vi "Vision Inspection Example.vi"(4 "Thread No.":u32, 5 "ProgramRef":refnum<vi>, 6 "Thread Mod Recive":refnum<queue>[](array[refnum]), 7 "ThreadsQueue":refnum<queue>[](array[refnum]), 8 "ThreadInfoIN":T1, 10 "StackIn":cluster{"Program":i32, "Prog Index":i32}[](array[cluster]), 11 "PrameterS":string) -> (0 "ThreadInfoOUT":T1, 2 "StackOut":cluster{"Program":i32, "Prog Index":i32}[](array[cluster]), 3 "ErrorCode":string)   [LabVIEW 2020]
uses:
  <vilib>/vision/Measure.llb/Edge Options.ctl
  <vilib>/vision/Measure.llb/Edge Polarity.ctl
  <vilib>/vision/Image Controls.llb/IMAQ Image.ctl
  <vilib>/vision/NI_Vision_Development_Module.lvlib
panel:
  in  "ResetPattern?":bool=TRUE
  out "DeltaAngle":sgl
  out "DeltaXY":cluster{"X":sgl, "Y":sgl}
  out "Angle":sgl=-46.475883
  out "CenterDL":cluster{"X":sgl, "Y":sgl}
  out "CenterUR":cluster{"X":sgl, "Y":sgl}
  in  "IMAQ?":bool=TRUE
  out "ROI Offset":cluster{"x":sgl, "y":sgl}
  out "FindCenter?":bool
  out "CenterPattern":T2(plugin-control)
  out "Pattern":T2(plugin-control)
  in  "SettingData":T5 {"FindCircleConfig"."Search  Direction" items=["Outside to Inside", "Inside to Outside"]; "FindCircleConfig"."Edge Options"."Edge Polarity" items=["All Edges", "Rising Edges", "Falling Edges"]; "FindCircleConfig"."Edge Options"."Minimum Edge Strength" format="%.2f"; "FindCircleConfig"."Edge Options"."Width" step=2; "FindCircleConfig"."Edge Options"."Kernel Size" step=2; "Range"."Maximum" format="%.2f"; "Range"."Minimum" format="%.2f"; "PatternCenter"."y" format="%.2f"; "PatternCenter"."x" format="%.2f"; "Algorithm" items=["All", "Low Discrepancy Sampling", "Grayscale Value Pyramid", "Gradients Pyramid"]}
  out "Test":T2(plugin-control)
  in  "Operation":enum16{"Setting", "Inspect"}(ring)=enum."Inspect"
  in  "ImagePath":path=path "D:/Project/V-KeyBoard Link Check/G3.png"
  # "ROI[0]: FindCenter"
  # "ROI[1]: Gap_up1"
  # "ROI[2]: Gap_up2"
  # "ROI[3]: Link_In1"
  # "ROI[4]: Link_In2"
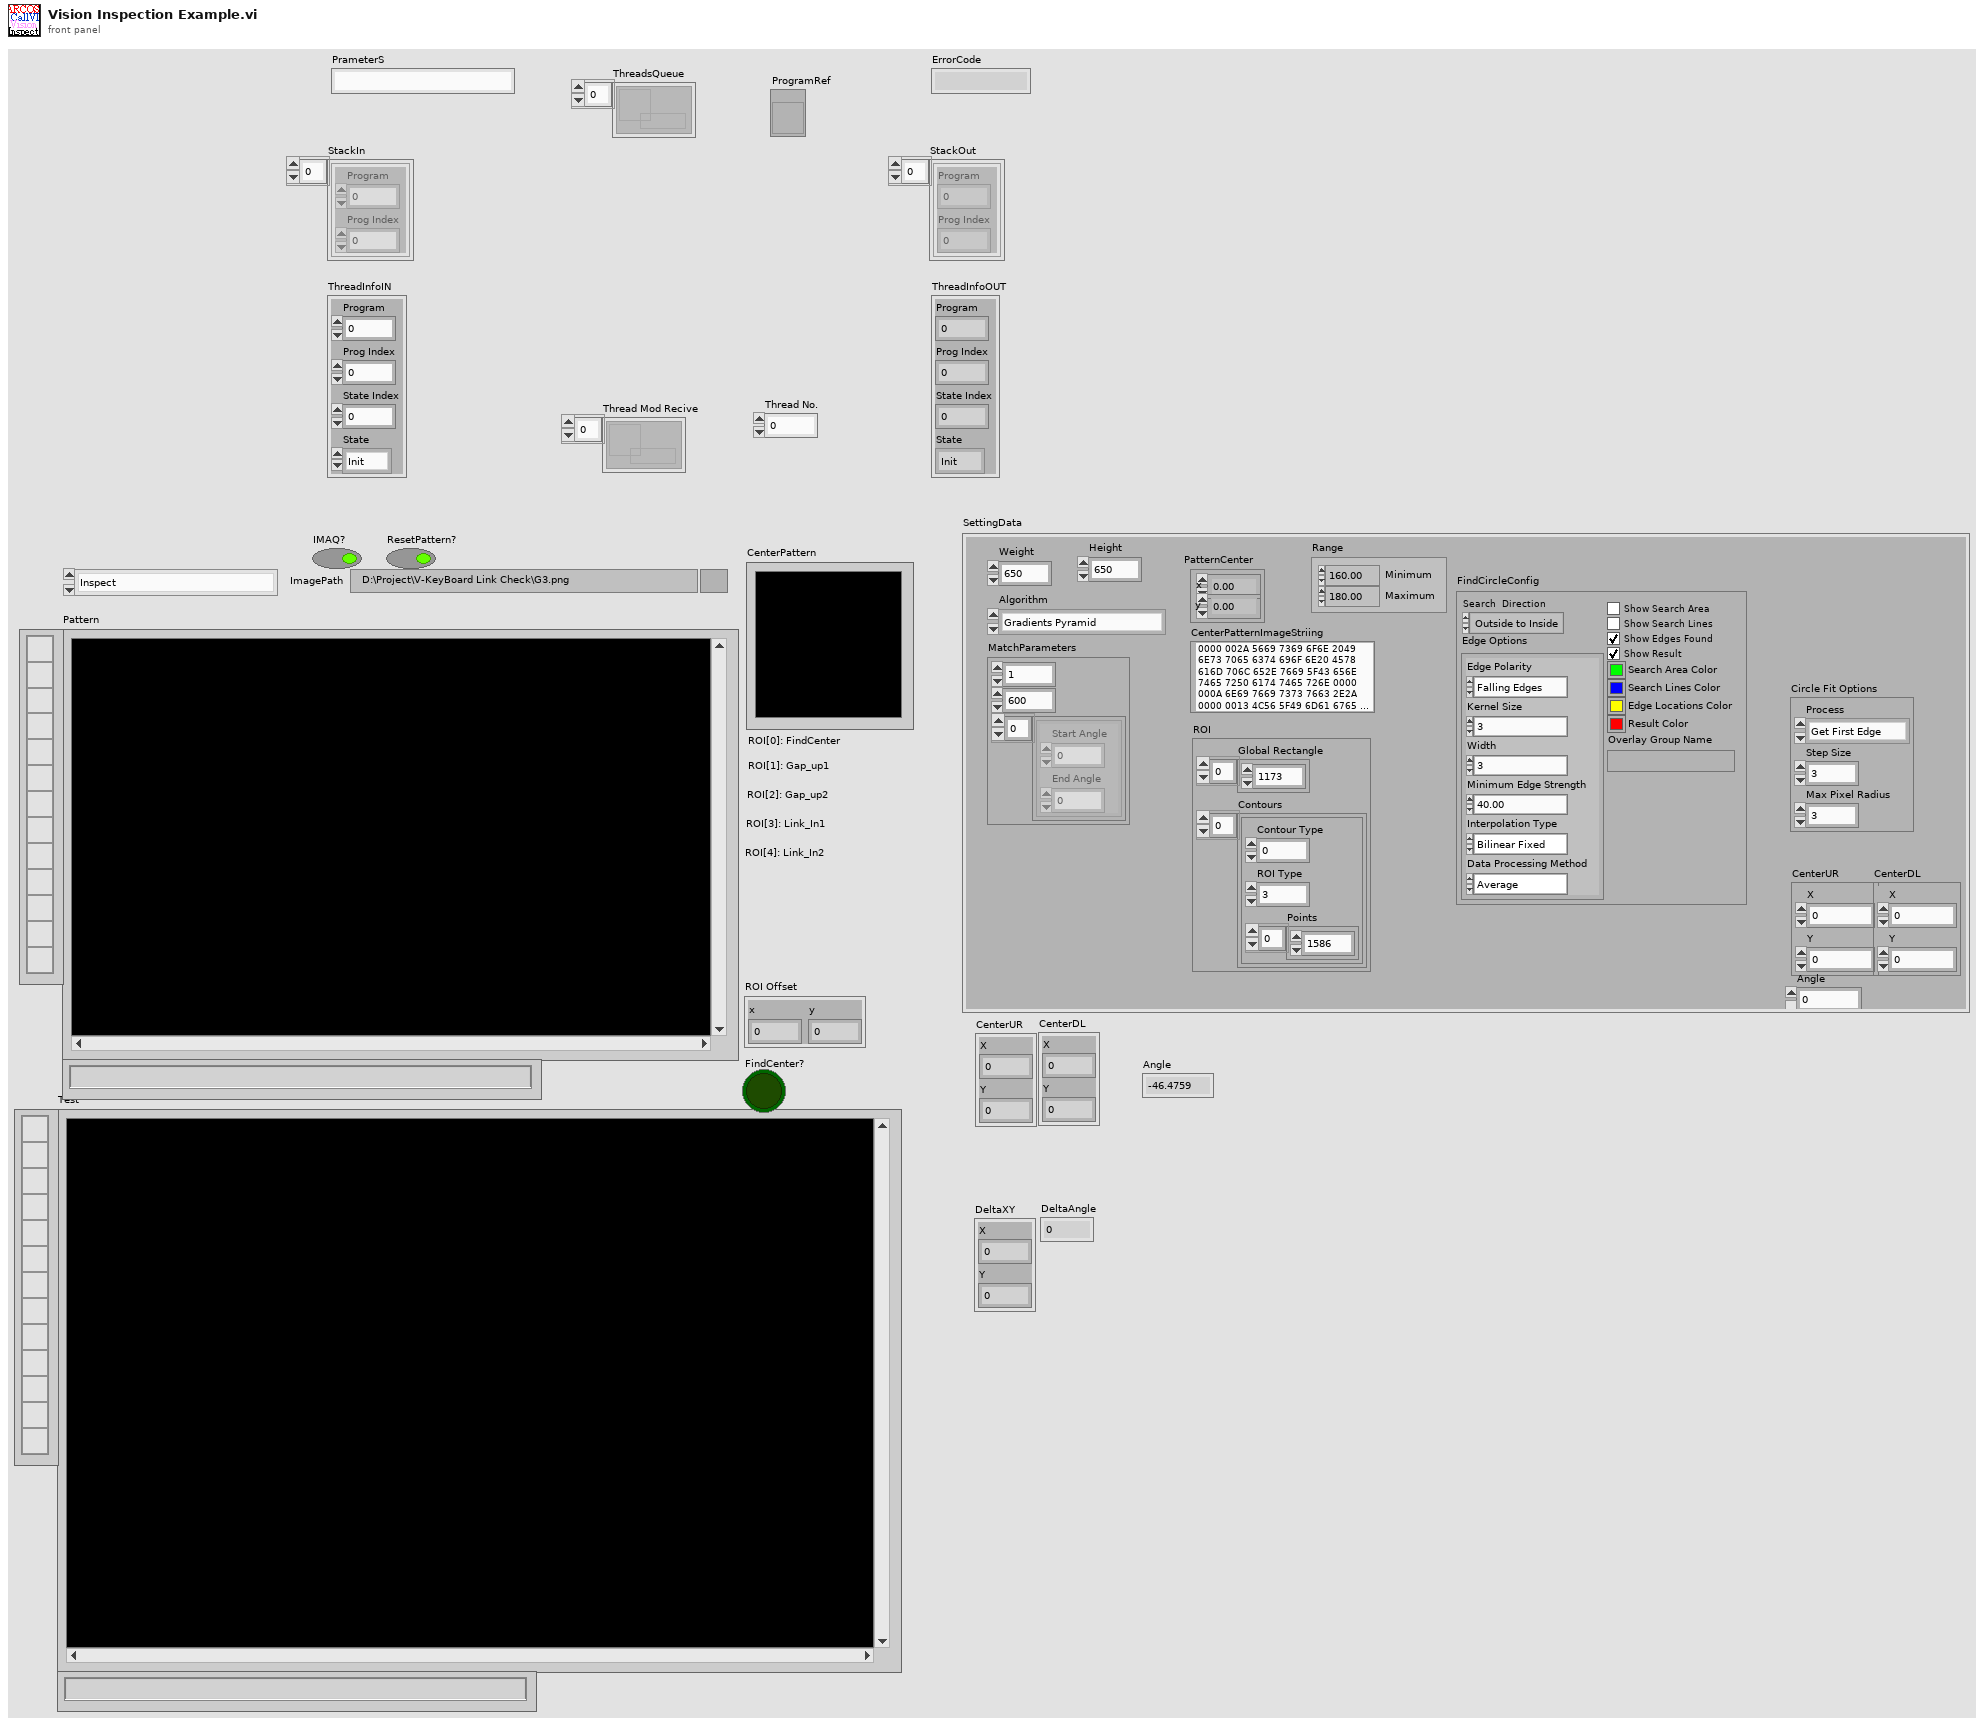
[diagram p1: front panel]
types:
  T1 = cluster{"Program":i32, "Prog Index":i32, "State Index":i32, "State":enum16{"Init", "Idle", "Auto Start", "Auto Running", "Step Start", "Step Running", "Suspend", "Restart", "Stop", "Reset"}}
  T2 = typedef "IMAQ Image.ctl" = refnum<image>
  T3 = typedef "Edge Options.ctl" = cluster{"Edge Polarity":T4, "Kernel Size":u32, "Width":u32, "Minimum Edge Strength":sgl, "Interpolation Type":enum32{"Zero Order", "Bilinear", "Quadratic", "Cubic", "Bilinear Fixed"}, "Data Processing Method":enum32{"Average", "Median"}}
  T4 = typedef "Edge Polarity.ctl" = u32
  T5 = cluster{"Weight":i32, "Height":i32, "MatchParameters":cluster{"Number of Matches Requested":i32, "Minimum Match Score":sgl, "Angle Ranges":cluster{"Start Angle":sgl, "End Angle":sgl}[]}, "Algorithm":i32, "CenterPatternImageStriing":string, "PatternCenter":cluster{"x":sgl, "y":sgl}, "ROI":cluster{"Global Rectangle":i32[], "Contours":cluster{"Contour Type":u32, "ROI Type":u32, "Points":i32[]}[]}, "Range":cluster{"Minimum":sgl, "Maximum":sgl}, "FindCircleConfig":cluster{"Search  Direction":u32, "Edge Options":T3, "Show Search Area":bool, "Show Search Lines":bool, "Show Edges Found":bool, "Show Result":bool, "Search Area Color":u32, "Search Lines Color":u32, "Edge Locations Color":u32, "Result Color":u32, "Overlay Group Name":string}, "Circle Fit Options":cluster{"Process":enum16{"Get First Edge", "Get First + Last Edge", "Get All Edges", "Get Best Edge"}, "Step Size":dbl, "Max Pixel Radius":i32}, "CenterUR":cluster{"X":sgl, "Y":sgl}, "CenterDL":cluster{"X":sgl, "Y":sgl}, "Angle":sgl}
  T6 = typedef "Image Type" = u32
  T7 = cluster{"Number of Matches Requested":i32, "Minimum Match Score":sgl, "Angle Ranges":cluster{"Start Angle":sgl, "End Angle":sgl}[]}
  T8 = cluster{"Search  Direction":u32, "Edge Options":T3, "Show Search Area":bool, "Show Search Lines":bool, "Show Edges Found":bool, "Show Result":bool, "Search Area Color":u32, "Search Lines Color":u32, "Edge Locations Color":u32, "Result Color":u32, "Overlay Group Name":string}
  T9 = cluster{"Process":enum16{"Get First Edge", "Get First + Last Edge", "Get All Edges", "Get Best Edge"}, "Step Size":dbl, "Max Pixel Radius":i32}
  T10 = cluster{"Global Rectangle":i32[], "Contours":cluster{"Contour Type":u32, "ROI Type":u32, "Points":i32[]}[]}
  T11 = cluster{"Contour Type":u32, "ROI Type":u32, "Points":i32[]}[]
  T12 = cluster{"Contour Type":u32, "ROI Type":u32, "Points":i32[]}
  T13 = cluster{"Position":cluster{"x":sgl, "y":sgl}, "Angle":sgl, "Scale":sgl, "Score":sgl, "Bounding Box":cluster{"x":sgl, "y":sgl}[]}[]
  T14 = cluster{"Position":cluster{"x":sgl, "y":sgl}, "Angle":sgl, "Scale":sgl, "Score":sgl, "Bounding Box":cluster{"x":sgl, "y":sgl}[]}
  T15 = cluster{"Center (Pixels)":cluster{"X":sgl, "Y":sgl}, "Radius (Pixels)":dbl, "Center (Real-World)":cluster{"X":sgl, "Y":sgl}, "Radius (Real-World)":dbl, "Roundness (Real-World)":dbl, "Average Strength":dbl, "Average SNR (dB)":dbl}
  T16 = cluster{"Origin":cluster{"X":sgl, "Y":sgl}, "Angle (deg)":sgl, "Axis Reference":u32}
  T17 = cluster{"ID":enum32{"External", "Internal"}, "Type":u32, "Coordinates":i32[]}[]
  T18 = cluster{"ID":enum32{"External", "Internal"}, "Type":u32, "Coordinates":i32[]}
  T19 = typedef "ROI Descriptor" = cluster{"Global Rectangle":i32[], "Contours":cluster{"ID":enum32{"External", "Internal"}, "Type":u32, "Coordinates":i32[]}[]}
  T20 = enum16{"Init", "Idle", "Auto Start", "Auto Running", "Step Start", "Step Running", "Suspend", "Restart", "Stop", "Reset"}
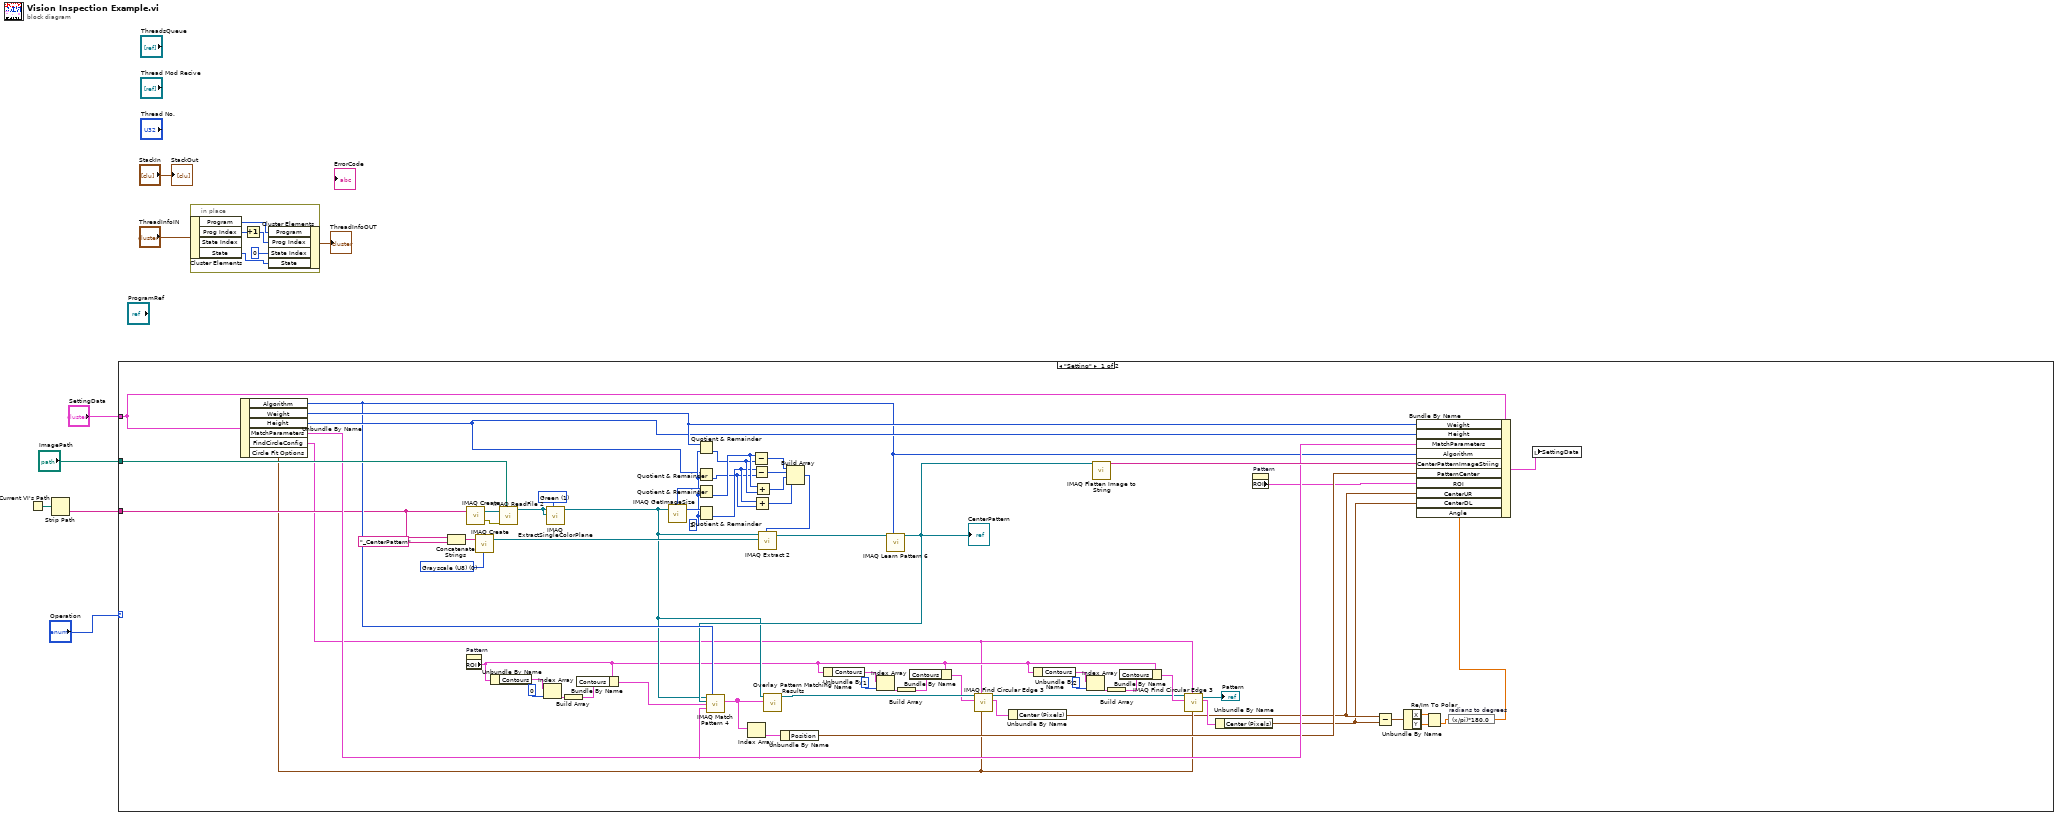
[diagram p0: block diagram]
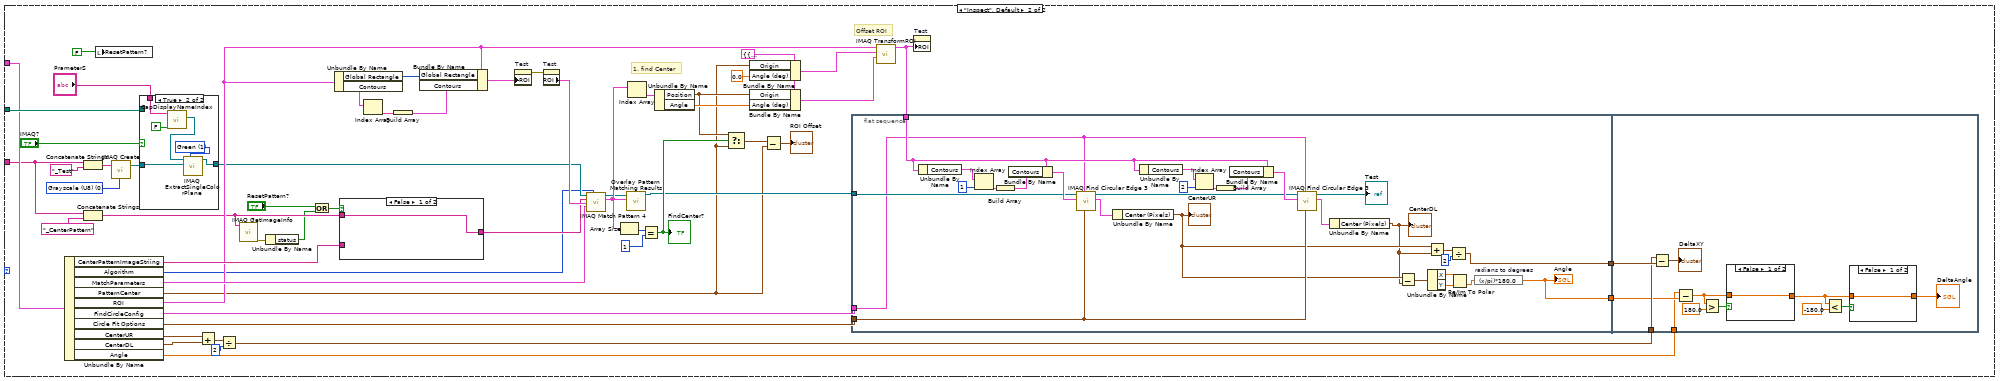
[diagram p2: hidden frame]
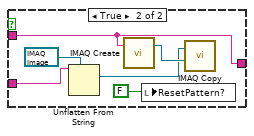
[diagram p3: hidden frame]
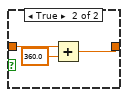
[diagram p4: hidden frame]
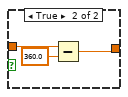
[diagram p5: hidden frame]
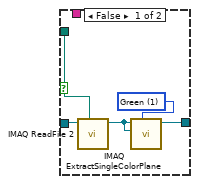
[diagram p6: hidden frame]
diagram:
  n1 = Current VI's Path() -> (path=w7:path)
  n2 = Strip Path(path=w7) -> (name=w6:string)  [unwired: 1 out]
  n3 = case shown="\"Setting\"" "Operation" {
    tunnel: w6 -> [w44 w90]
    tunnel: "ImagePath" -> [w57 w130]
    tunnel: "SettingData" -> [w56 w125]
    frame "Setting" {
      w35 = 1 items=["Red", "Green", "Blue", "Hue", "Saturation", "Luminance", "Value", "Intensity"] ("Color Plane")
      w58 = T6 0 items=["Grayscale (U8)", "Grayscale (I16)", "Grayscale (SGL)", "Complex (CSG)", "RGB (U32)", "HSL (U32)", "RGB (U64)", "Grayscale (U16)"] ("Image Type")
      w68 = 2 ("y")
      n4 = Unbundle By Name(w56) -> ("Algorithm"=w50:i32, "Weight"=w54:i32, "Height"=w53:i32, "MatchParameters"=w51:T7, "FindCircleConfig"=w20:T8, "Circle Fit Options"=w18:T9)
      n5 = Concatenate Strings(w44, "_CenterPattern" ("string")) -> (w71:string)
      n6 = property on="Pattern" class="ImageControl"() -> ("ROI"=w21:T10)  [unwired: 2 in, 2 out]
      n7 = call "IMAQ Create"("Image Name"=w44) -> ("New Image"=w73:T2, "error out"=w74:errorcluster)  [unwired: 4 in]
      n8 = call "IMAQ Create"("Image Name"=w71, "Image Type"=w58) -> ("New Image"=w38:T2)  [unwired: 3 in, 1 out]
      n9 = Unbundle By Name(w21) -> ("Contours"=w43:T11)
      n10 = call "IMAQ ReadFile 2"("File Path"=w57, "error in (no error)"=w74, "Image"=w73) -> ("Image Out"=w36:T2)  [unwired: 4 in, 4 out]
      n11 = Index Array(array=w43, index=0) -> (element=w41:T12)
      n12 = call "IMAQ ExtractSingleColorPlane"("Color Plane"=w35, "Image Dst"=w36, "Image Src"=w36) -> ("Image Dst Out"=w34:T2)  [unwired: 7 in, 1 out]
      n13 = Build Array(w41) -> (w40:T11)
      n14 = Bundle By Name(cluster=w21, "Contours"=w40) -> (w39:T10)
      n15 = call "IMAQ GetImageSize"("Image"=w34) -> ("Y Resolution"=w69:i32, "X Resolution"=w70:i32)  [unwired: 3 in, 1 out]
      n16 = Quotient & Remainder(x=w53, y=w68) -> (floor(x/y)=w64:i32)  [unwired: 1 out]
      n17 = Quotient & Remainder(x=w54, y=w68) -> (floor(x/y)=w66:i32)  [unwired: 1 out]
      n18 = Quotient & Remainder(x=w70, y=w68) -> (floor(x/y)=w67:i32)  [unwired: 1 out]
      n19 = Quotient & Remainder(x=w69, y=w68) -> (floor(x/y)=w65:i32)  [unwired: 1 out]
      n20 = Subtract(x=w67, y=w66) -> (x-y=w63:i32)
      n21 = Subtract(x=w65, y=w64) -> (x-y=w62:i32)
      n22 = Add(x=w65, y=w64) -> (x+y=w60:i32)
      n23 = Add(x=w67, y=w66) -> (x+y=w61:i32)
      n24 = Build Array(w63, w62, w61, w60) -> (w59:i32[])
      n25 = call "IMAQ Extract 2"("Optional Rectangle"=w59, "Image Dst"=w38, "Image Src"=w34) -> ("Image Dst Out"=w37:T2)  [unwired: 7 in, 1 out]
      n26 = Unbundle By Name(w21) -> ("Contours"=w29:T11)
      n27 = Index Array(array=w29, index=1) -> (element=w31:T12)
      n28 = call "IMAQ Learn Pattern 6"("Image"=w37, "Algorithm"=w50) -> ("Template Image Out"=w49:T2)  [unwired: 11 in, 2 out]
      "CenterPattern" <- w49
      n29 = call "IMAQ Match Pattern 4"("Image"=w34, "Algorithm"=w50, "Template Image"=w49, "ROI Descriptor"=w39, "Parameters"=w51) -> ("Matches (pixel)"=w48:T13)  [unwired: 6 in, 4 out]
      n30 = Index Array(array=w48) -> (element=w47:T14)  [unwired: 1 in]
      n31 = call "Overlay Pattern Matching Results.vi"("Matches"=w48, "Image"=w34) -> ("Image Out"=w33:T2)  [unwired: 8 in, 1 out]
      n32 = Unbundle By Name(w47) -> ("Position"=w46:cluster{"x":sgl, "y":sgl})
      n33 = Build Array(w31) -> (w32:T11)
      n34 = Bundle By Name(cluster=w21, "Contours"=w32) -> (w28:T10)
      n35 = call "IMAQ Find Circular Edge 3"("Circle Fit Options"=w18, "Options"=w20, "ROI Descriptor"=w28, "Image"=w33) -> ("Fitted Circle"=w17:T15, "Image Out"=w22:T2)  [unwired: 3 in, 3 out]
      n36 = Unbundle By Name(w17) -> ("Center (Pixels)"=w15:cluster{"X":sgl, "Y":sgl})
      n37 = Unbundle By Name(w21) -> ("Contours"=w26:T11)
      n38 = Index Array(array=w26, index=2) -> (element=w24:T12)
      n39 = call "IMAQ Flatten Image to String"("Image"=w49) -> ("Data String"=w55:string)  [unwired: 9 in, 1 out]
      n40 = Build Array(w24) -> (w23:T11)
      n41 = Bundle By Name(cluster=w21, "Contours"=w23) -> (w27:T10)
      n42 = call "IMAQ Find Circular Edge 3"("Circle Fit Options"=w18, "Options"=w20, "ROI Descriptor"=w27, "Image"=w22) -> ("Fitted Circle"=w16:T15, "Image Out"=→"Pattern":T2)  [unwired: 3 in, 3 out]
      n43 = Unbundle By Name(w16) -> ("Center (Pixels)"=w14:cluster{"X":sgl, "Y":sgl})
      n44 = property on="Pattern" class="ImageControl"() -> ("ROI"=w45:T10)  [unwired: 2 in, 2 out]
      n45 = Subtract(x=w15, y=w14) -> (x-y=w13:cluster{"X":sgl, "Y":sgl})
      n46 = Unbundle By Name(w13) -> ("X"=w12:sgl, "Y"=w11:sgl)
      n47 = Re/Im To Polar(2:w11, 3:w12) -> (0:w10:sgl)  [unwired: 1 out]
      n48 = expression code="(x/pi)*180.0" "radians to degrees"(w10) -> (w9:sgl)
      n49 = Bundle By Name(cluster=w56, "Weight"=w54, "Height"=w53, "MatchParameters"=w51, "Algorithm"=w50, "CenterPatternImageStriing"=w55, "PatternCenter"=w46, "ROI"=w45, "CenterUR"=w15, "CenterDL"=w14, "Angle"=w9) -> (w52:T5)
      n50 = local write "SettingData"(w52) -> ()
    }
    frame "Inspect", Default {
      w92 = T6 0 items=["Grayscale (U8)", "Grayscale (I16)", "Grayscale (SGL)", "Complex (CSG)", "RGB (U32)", "HSL (U32)", "RGB (U64)", "Grayscale (U16)"] ("Image Type")
      w86 = T16 {"Origin"={"X"=0.0, "Y"=0.0}, "Angle (deg)"=0.0, "Axis Reference"=0} ("Base Reference")
      # "Offset ROI"
      # "1. find Center"
      n51 = Unbundle By Name(w125) -> ("CenterPatternImageStriing"=w127:string, "Algorithm"=w81:i32, "MatchParameters"=w128:T7, "PatternCenter"=w85:cluster{"x":sgl, "y":sgl}, "ROI"=w112:T10, "FindCircleConfig"=w103:T8, "Circle Fit Options"=w102:T9, "CenterUR"=w99:cluster{"X":sgl, "Y":sgl}, "CenterDL"=w98:cluster{"X":sgl, "Y":sgl}, "Angle"=w94:sgl)
      n52 = Concatenate Strings(w90, "_Test" ("string")) -> (w93:string)
      n53 = Concatenate Strings(w90, "_CenterPattern" ("string")) -> (w80:string)
      n54 = local write "ResetPattern?"(FALSE ("Reset?")) -> ()
      n55 = call "IMAQ Create"("Image Name"=w93, "Image Type"=w92) -> ("New Image"=w89:T2)  [unwired: 3 in, 1 out]
      n56 = case shown="True" "IMAQ?" {
        tunnel: w130 -> [w190 _]
        tunnel: [w187 w194] -> w108
        tunnel: w89 -> [w186 w195]
        tunnel: "PrameterS" -> [_ w191]
        frame False {
          w189 = 1 items=["Red", "Green", "Blue", "Hue", "Saturation", "Luminance", "Value", "Intensity"] ("Color Plane")
          n57 = call "IMAQ ReadFile 2"("File Path"=w190, "Image"=w186) -> ("Image Out"=w188:T2)  [unwired: 5 in, 4 out]
          n58 = call "IMAQ ExtractSingleColorPlane"("Color Plane"=w189, "Image Dst"=w188, "Image Src"=w188) -> ("Image Dst Out"=w187:T2)  [unwired: 7 in, 1 out]
        }
        frame True {
          w196 = 1 items=["Red", "Green", "Blue", "Hue", "Saturation", "Luminance", "Value", "Intensity"] ("Color Plane")
          n59 = call "CapDisplayNameIndex.vi"("Init?"=FALSE, "CamName"=w191) -> ("IMAQ"=w192:T2)  [unwired: 3 in, 3 out]
          n60 = call "IMAQ ExtractSingleColorPlane"("Color Plane"=w196, "Image Dst"=w195, "Image Src"=w192) -> ("Image Dst Out"=w194:T2)  [unwired: 7 in, 1 out]
        }
      }
      n61 = Add(x=w99, y=w98) -> (x+y=w100:cluster{"X":sgl, "Y":sgl})
      n62 = Divide(x=w100, y=2) -> (x/y=w95:cluster{"X":sgl, "Y":sgl})
      n63 = call "IMAQ GetImageInfo"("Image"=w80) -> ("error out"=w79:errorcluster)  [unwired: 3 in, 7 out]
      n64 = Unbundle By Name(w79) -> ("status"=w76:bool)
      n65 = Or(x="ResetPattern?", y=w76) -> (x .or. y?=w78:bool)
      n66 = Unbundle By Name(w112) -> ("Global Rectangle"=w118:i32[], "Contours"=w121:T11)
      n67 = case shown="False" w78 {
        tunnel: w127 -> [_ w137]
        tunnel: [w131 w134] -> w106
        tunnel: w80 -> [w131 w134]
        frame False {
        }
        frame True {
          n68 = Unflatten From String(type=T2 refnum ("New Image"), binary string=w137) -> (value=w132:T2)  [unwired: 3 in, 2 out]
          n69 = call "IMAQ Create"("Image Name"=w134) -> ("New Image"=w133:T2)  [unwired: 4 in, 1 out]
          n70 = local write "ResetPattern?"(FALSE ("ResetPattern?")) -> ()
          n71 = call "IMAQ Copy"("Image Dst"=w133, "Image Src"=w132) -> ()  [unwired: 4 in, 2 out]
        }
      }
      n72 = Index Array(array=w121) -> (element=w120:T12)  [unwired: 1 in]
      n73 = Build Array(w120) -> (w119:T11)
      n74 = Bundle By Name(cluster=w112, "Global Rectangle"=w118, "Contours"=w119) -> (w117:T10)
      n75 = property on="Test" class="ImageControl"("ROI"=w117) -> (error out=w116:errorcluster)  [unwired: 2 in, 1 out]
      n76 = property on="Test" class="ImageControl"(error in=w116) -> ("ROI"=w115:T10)  [unwired: 1 in, 2 out]
      n77 = call "IMAQ Match Pattern 4"("Image"=w108, "Algorithm"=w81, "Template Image"=w106, "ROI Descriptor"=w115, "Parameters"=w128) -> ("Image (duplicate)"=w111:T2, "Matches (pixel)"=w124:T13)  [unwired: 6 in, 3 out]
      n78 = Array Size(array=w124) -> (size(s)=w123:i32)
      n79 = call "Overlay Pattern Matching Results.vi"("Matches"=w124, "Image"=w111) -> ("Image Out"=w104:T2)  [unwired: 8 in, 1 out]
      n80 = Index Array(array=w124) -> (element=w126:T14)  [unwired: 1 in]
      n81 = Equal?(x=w123, y=1) -> (x = y?=w110:bool)
      "FindCenter?" <- w110
      n82 = Unbundle By Name(w126) -> ("Position"=w87:cluster{"x":sgl, "y":sgl}, "Angle"=w88:sgl)
      n83 = Select(t=w87, s=w110, f=w85) -> (s? t:f=w109:cluster{"x":sgl, "y":sgl})
      n84 = Bundle By Name(cluster=w86, "Origin"=w85, "Angle (deg)"=sgl 0.0) -> (w83:T16)
      n85 = Bundle By Name(cluster=w86, "Origin"=w87, "Angle (deg)"=w88) -> (w113:T16)
      n86 = Subtract(x=w109, y=w85) -> (x-y=→"ROI Offset":cluster{"x":sgl, "y":sgl})
      n87 = flat-sequence {
        tunnel: w105 -> [w152]
        tunnel: w104 -> [w151]
        tunnel: w103 -> [w149]
        tunnel: w102 -> [w150]
        tunnel: [w139] -> w97
        tunnel: [w138] -> w96
        tunnel: w97 -> [w177]
        tunnel: w96 -> [w175]
        tunnel: w95 -> [w176]
        tunnel: w94 -> [w174]
        frame #0 {
          n88 = Unbundle By Name(w152) -> ("Contours"=w163:T17)
          n89 = Index Array(array=w163, index=1) -> (element=w164:T18)
          n90 = Build Array(w164) -> (w165:T17)
          n91 = Bundle By Name(cluster=w152, "Contours"=w165) -> (w162:T19)
          n92 = call "IMAQ Find Circular Edge 3"("Circle Fit Options"=w150, "Options"=w149, "ROI Descriptor"=w162, "Image"=w151) -> ("Fitted Circle"=w156:T15, "Image Out"=w157:T2)  [unwired: 3 in, 3 out]
          n93 = Unbundle By Name(w156) -> ("Center (Pixels)"=w143:cluster{"X":sgl, "Y":sgl})
          "CenterUR" <- w143
          n94 = Unbundle By Name(w152) -> ("Contours"=w160:T17)
          n95 = Index Array(array=w160, index=2) -> (element=w159:T18)
          n96 = Build Array(w159) -> (w158:T17)
          n97 = Bundle By Name(cluster=w152, "Contours"=w158) -> (w161:T19)
          n98 = call "IMAQ Find Circular Edge 3"("Circle Fit Options"=w150, "Options"=w149, "ROI Descriptor"=w161, "Image"=w157) -> ("Fitted Circle"=w155:T15, "Image Out"=→"Test":T2)  [unwired: 3 in, 3 out]
          n99 = Unbundle By Name(w155) -> ("Center (Pixels)"=w142:cluster{"X":sgl, "Y":sgl})
          "CenterDL" <- w142
          n100 = Subtract(x=w143, y=w142) -> (x-y=w147:cluster{"X":sgl, "Y":sgl})
          n101 = Unbundle By Name(w147) -> ("X"=w146:sgl, "Y"=w145:sgl)
          n102 = Add(x=w143, y=w142) -> (x+y=w141:cluster{"X":sgl, "Y":sgl})
          n103 = Divide(x=w141, y=2) -> (x/y=w139:cluster{"X":sgl, "Y":sgl})
          n104 = Re/Im To Polar(2:w145, 3:w146) -> (0:w144:sgl)  [unwired: 1 out]
          n105 = expression code="(x/pi)*180.0" "radians to degrees"(w144) -> (w138:sgl)
          "Angle" <- w138
        }
        frame #1 {
          n106 = Subtract(x=w176, y=w177) -> (x-y=→"DeltaXY":cluster{"X":sgl, "Y":sgl})
          n107 = Subtract(x=w174, y=w175) -> (x-y=w170:sgl)
          n108 = Greater?(x=w170, y=sgl 180.0) -> (0:w171:bool)
          n109 = case shown="False" w171 {
            tunnel: w170 -> [w182 w185]
            tunnel: [w182 w183] -> w167
            frame False {
            }
            frame True {
              n110 = Subtract(x=w185, y=sgl 360.0) -> (x-y=w183:sgl)
            }
          }
          n111 = Less?(x=w167, y=sgl -180.0) -> (x < y?=w168:bool)
          n112 = case shown="False" w168 {
            tunnel: w167 -> [w178 w181]
            tunnel: [w178 w179] -> w166
            frame False {
            }
            frame True {
              n113 = Add(x=w181, y=sgl 360.0) -> (x+y=w179:sgl)
            }
          }
          "DeltaAngle" <- w166
        }
      }
      n114 = call "IMAQ TransformROI"("New Reference"=w113, "Base Reference"=w83, "ROI Descriptor"=w112) -> ("ROI Descriptor out"=w105:T19)  [unwired: 7 in, 1 out]
      n115 = property on="Test" class="ImageControl"("ROI"=w105) -> ()  [unwired: 2 in, 2 out]
    }
  }
  n116 = in-place {
    n117 = in-place-cluster #1("ThreadInfoIN") -> ("Program"=w201:i32, "Prog Index"=w199:i32, "State"=w197:T20)  [unwired: 1 out]
    n118 = Increment(x=w199) -> (x+1=w200:i32)
    n119 = in-place-cluster #1("Program"=w201, "Prog Index"=w200, "State Index"=0, "State"=w197) -> (→"ThreadInfoOUT":T1)
  }
  "StackOut" <- "StackIn"
